vi "GetEncType.vi"(8 "错误输入（无错误）":errorcluster, 11 "编码器序号":i32) -> (0 "错误输出":errorcluster, 3 "返回值":u8)   [LabVIEW 2014]
uses:
  X86Dll/ZXUTConfigMgr.dll
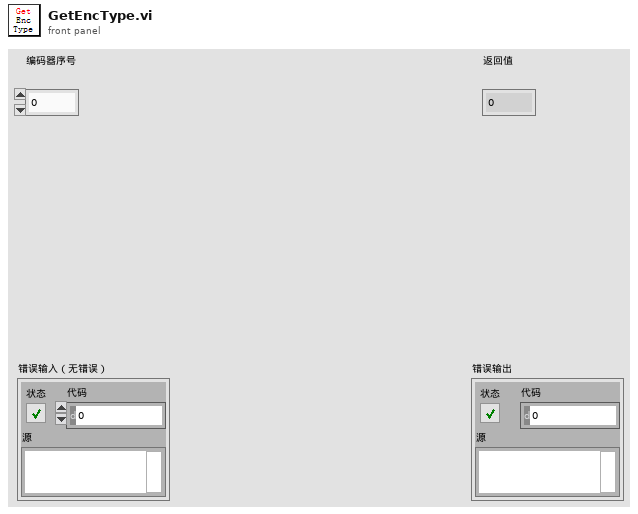
[diagram p1: front panel]
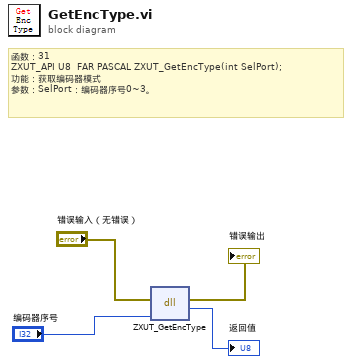
[diagram p0: block diagram]
diagram:
  # "函数：31\nZXUT_API U8\t\tFAR PASCAL ZXUT_GetEncType(int SelPort);\n功能：获取编码器模式\n参数：SelPort：编码器序号0~3。"
  n1 = dll-call lib="D:/Software/Utrasonic on-line monitoring/X86Dll/ZXUTConfigMgr.dll" fn="ZXUT_GetEncType"(error in="错误输入（无错误）", "SelPort"="编码器序号") -> (error out=→"错误输出":errorcluster, "返回值"=→"返回值":u8)  [unwired: 3 in, 1 out]
